vi "Host - Thruster Cmd encode (SubVI).vi"(7 "Address":u16=111 format="%.0x", 11 "Thruster ctrl":i16 min=-25 max=25) -> (3 "cmd Array":u32[](array[numeric]))   [LabVIEW 2021]
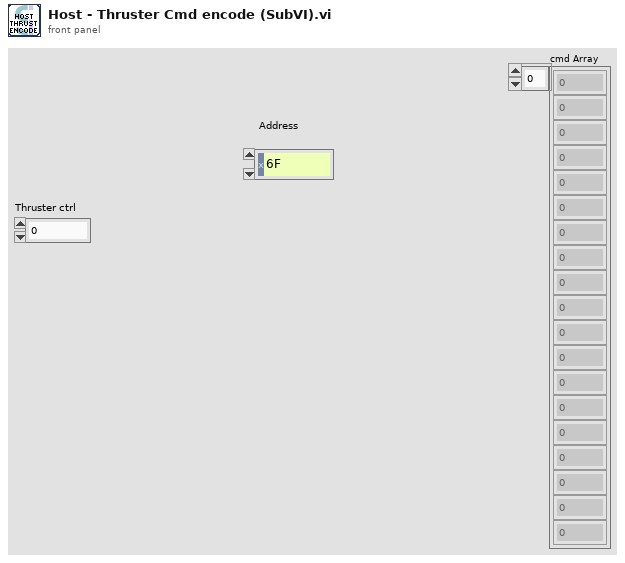
[diagram p1: front panel]
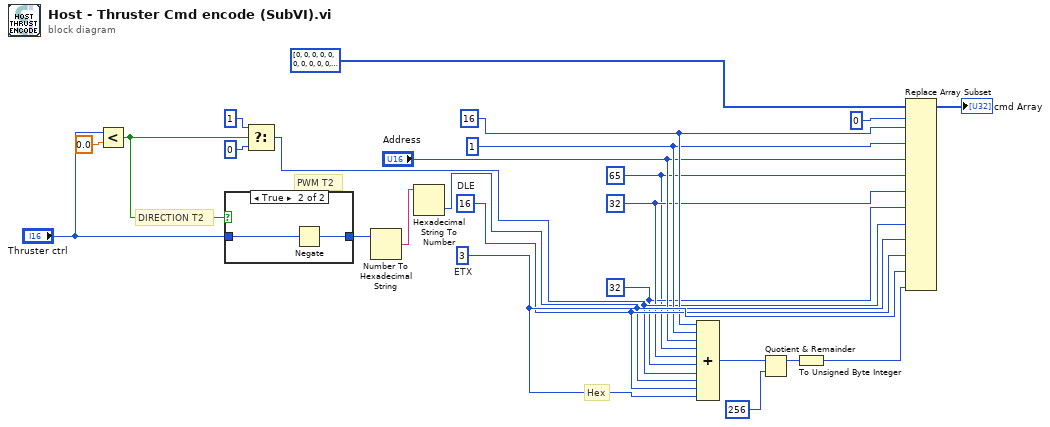
[diagram p0: block diagram]
diagram:
  w2 = u16 65 ("DB1")
  w3 = u16 32 ("DB2")
  w4 = u16 32 ("DB1")
  w21 = u16 1 ("SOH")
  w22 = u16 16 ("DLE 2")
  w23 = u16 16  # DLE
  w24 = u16 3  # ETX
  # "Hex"
  # "DIRECTION T2"
  # "PWM T2"
  n1 = Less?(x="Thruster ctrl", y=0.0) -> (x < y?=w16:bool)
  n2 = case shown="True" w16 {
    tunnel: "Thruster ctrl" -> [w25 w27]
    tunnel: [w25 w26] -> w12
    frame False {
    }
    frame True {
      n3 = Negate(x=w27) -> (-x=w26:i16)
    }
  }
  n4 = Select(t=u8 1, s=w16, f=u8 0) -> (s? t:f=w15:u8)
  n5 = Number To Hexadecimal String(2:w12) -> (0:w13:string)  [unwired: 1 in]
  n6 = Hexadecimal String To Number(string=w13) -> (number=w11:u32)  [unwired: 2 in, 1 out]
  n7 = Compound Arithmetic op=ADD(w22, w21, "Address", w2, w4, w3, w15, w11, w23, w24) -> (w7:u32)
  n8 = Quotient & Remainder(x=w7, y=u16 256) -> (x-y*floor(x/y)=w8:u32)  [unwired: 1 out]
  n9 = To Unsigned Byte Integer(number=w8) -> (unsigned 8bit integer=w5:u8)
  n10 = Replace Array Subset(array=u32[] [0, 0, 0, 0, 0, 0, 0, 0, 0, 0, 0] ("output array"), new element #1=w22, index #1=0 ("index"), new element #2=w21, new element #3="Address", new element #4=w2, new element #5=w4, new element #6=w3, new element #7=w15, new element #8=w11, new element #9=w23, new element #10=w24, new element #11=w5) -> (→"cmd Array":u32[])  [unwired: 10 in]
